vi "HMI Command.vi"(9 "RIO CMD":dbl min=0.0 max=100.0 step=0.1 format="%#.2f", 10 "HMI CMD":dbl, 11 "Prev CMD":dbl) -> (2 "Boolean":bool, 3 "CMD OUT":dbl)   [LabVIEW 2019]
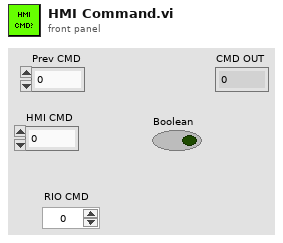
[diagram p1: front panel]
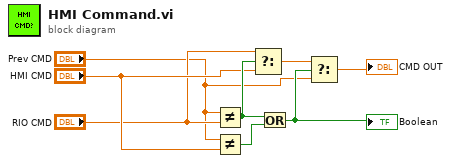
[diagram p0: block diagram]
diagram:
  n1 = Not Equal?(x="Prev CMD", y="RIO CMD") -> (x != y?=w8:bool)
  n2 = Not Equal?(x="Prev CMD", y="HMI CMD") -> (x != y?=w7:bool)
  n3 = Select(t="RIO CMD", s=w8, f="HMI CMD") -> (s? t:f=w4:dbl)
  n4 = Or(x=w8, y=w7) -> (x .or. y?=w3:bool)
  "Boolean" <- w3
  n5 = Select(t=w4, s=w3, f="Prev CMD") -> (s? t:f=→"CMD OUT":dbl)
